vi "SelectCommand.vi"(6 "ENABLE LASER":bool=TRUE, 7 "SelectCommand":string(combo)="CharacterString", 8 "error in (no error)":errorcluster, 9 "NewString":string="Prueba", 10 "BLOK (000)":string="000", 11 "PROGRAM (0000)":string="0000") -> (0 "error out":errorcluster, 3 "Command":string="\"\"")   [LabVIEW 2018]
doc: "This VI Construct the command with the correct syntax, add new commands if is necessary here."
panel:
  in  "Counter ID":string="0"
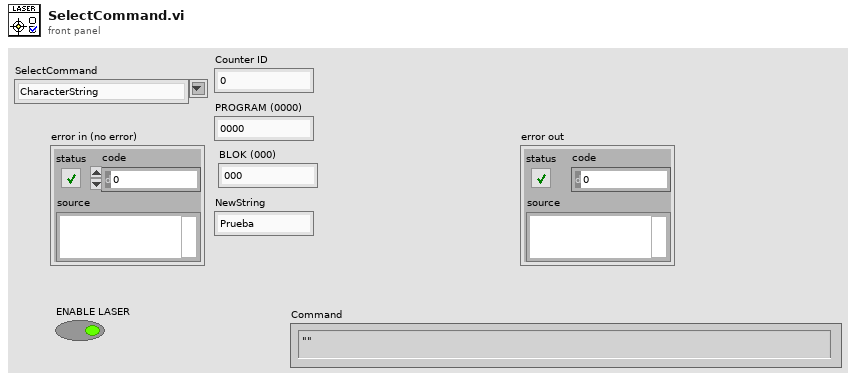
[diagram p1: front panel]
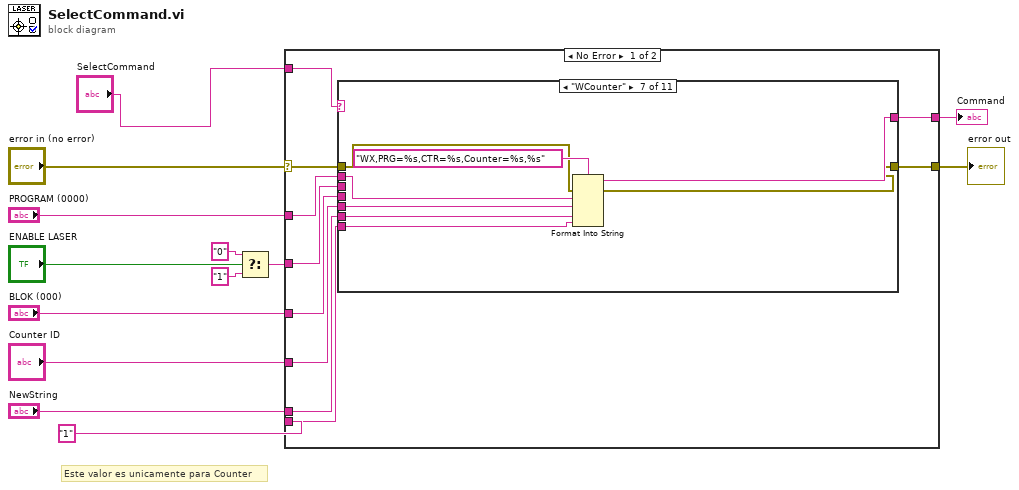
[diagram p0: block diagram]
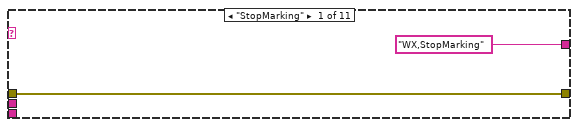
[diagram p2: hidden frame]
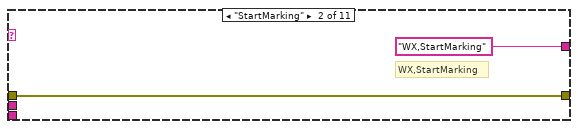
[diagram p3: hidden frame]
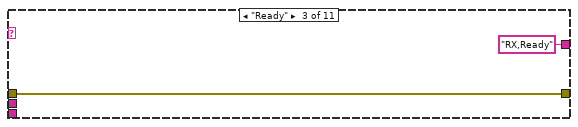
[diagram p4: hidden frame]
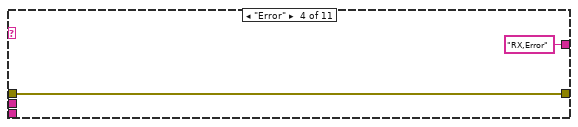
[diagram p5: hidden frame]
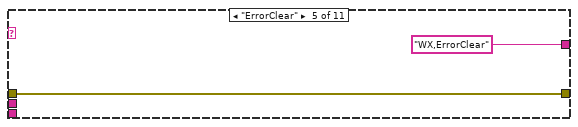
[diagram p6: hidden frame]
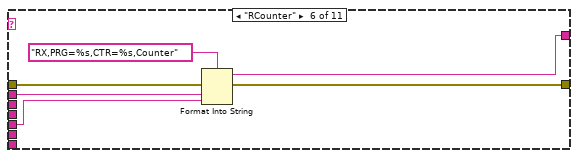
[diagram p7: hidden frame]
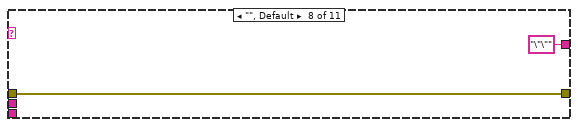
[diagram p8: hidden frame]
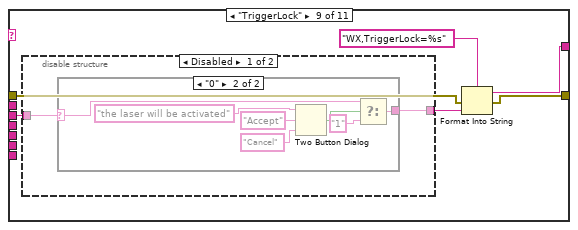
[diagram p9: hidden frame]
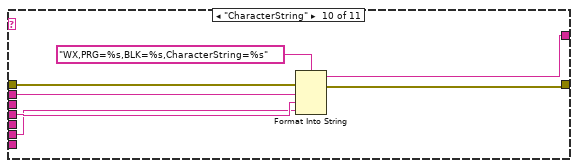
[diagram p12: hidden frame]
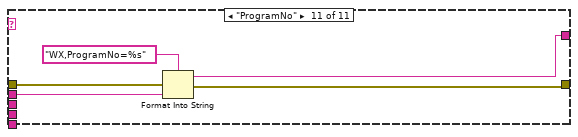
[diagram p13: hidden frame]
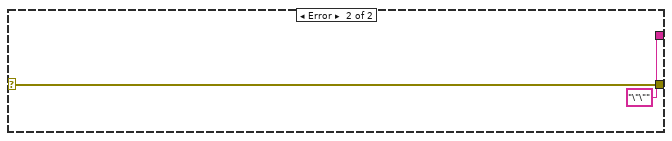
[diagram p14: hidden frame]
diagram:
  # "Este valor es unicamente para Counter"
  n1 = Select(t="0" ("WK or RX"), s="ENABLE LASER", f="1") -> (s? t:f=w4:string)
  n2 = case shown="No Error" "error in (no error)" {
    selector: "error in (no error)" -> [w16 w80]
    tunnel: [w15 w80] -> w12
    tunnel: [w23 "\"\"" ("CommandSelected")] -> w11
    tunnel: "PROGRAM (0000)" -> [w22 _]
    tunnel: "BLOK (000)" -> [w21 _]
    tunnel: "NewString" -> [w20 _]
    tunnel: w4 -> [w19 _]
    tunnel: "Counter ID" -> [w18 _]
    tunnel: "1" ("input 4") -> [w17 _]
    tunnel: "SelectCommand" -> [w14 _]
    frame No Error {
      n3 = case shown="\"WCounter\"" w14 {
        tunnel: ["WX,StopMarking" ("CommandSelected") "WX,StartMarking" ("CommandSelected") "RX,Ready" ("CommandSelected") "RX,Error" ("CommandSelected") "WX,ErrorClear" ("CommandSelected") w38 w46 "\"\"" ("CommandSelected") w55 w69 w77] -> w23
        tunnel: w22 -> [_ _ _ _ _ w37 w45 _ _ w72 w76]
        tunnel: w21 -> [_ _ _ _ _ _ _ _ _ w71 _]
        tunnel: w20 -> [_ _ _ _ _ _ w43 _ _ w70 _]
        tunnel: w19 -> [_ _ _ _ _ _ _ _ w54 _ _]
        tunnel: w18 -> [_ _ _ _ _ w36 w44 _ _ _ _]
        tunnel: w17 -> [_ _ _ _ _ _ w40 _ _ _ _]
        tunnel: w16 -> [w24 w26 w28 w30 w32 w35 w42 w48 w51 w68 w75]
        tunnel: [w24 w26 w28 w30 w32 w34 w41 w48 w50 w67 w74] -> w15
        frame "StopMarking" {
        }
        frame "StartMarking" {
          # "WX,StartMarking"
        }
        frame "Ready" {
        }
        frame "Error" {
        }
        frame "ErrorClear" {
        }
        frame "RCounter" {
          n4 = Format Into String(format string="RX,PRG=%s,CTR=%s,Counter", error in=w35, w37, w36) -> (resulting string=w38:string, error out=w34:errorcluster)  [unwired: 1 in]
        }
        frame "WCounter" {
          n5 = Format Into String(format string="WX,PRG=%s,CTR=%s,Counter=%s,%s", error in=w42, w45, w44, w43, w40) -> (resulting string=w46:string, error out=w41:errorcluster)  [unwired: 1 in]
        }
        frame "", Default {
        }
        frame "TriggerLock" {
          n6 = disable-structure shown="Disabled" {
            disable-tunnel: w54 -> [w57 w66]
            disable-tunnel: [w56 w66] -> w53
            frame Disabled {
              n7 = case shown="\"0\"" w57 {
                selector: w57 -> [w58 w61]
                tunnel: [w58 w60] -> w56
                frame "1", Default {
                }
                frame "0" {
                  n8 = Two Button Dialog(message="the laser will be activated", 1:"Cancel" ("F button name (\"Cancel\")"), 2:"Accept" ("T button name (\"OK\")")) -> (T button?=w62:bool)
                  n9 = Select(t=w61, s=w62, f="1") -> (s? t:f=w60:string)
                }
              }
            }
            frame Enabled {
            }
          }
          n10 = Format Into String(format string="WX,TriggerLock=%s", error in=w51, w53) -> (resulting string=w55:string, error out=w50:errorcluster)  [unwired: 1 in]
        }
        frame "CharacterString" {
          n11 = Format Into String(format string="WX,PRG=%s,BLK=%s,CharacterString=%s", error in=w68, w72, w71, w70) -> (resulting string=w69:string, error out=w67:errorcluster)  [unwired: 1 in]
        }
        frame "ProgramNo" {
          n12 = Format Into String(format string="WX,ProgramNo=%s", error in=w75, w76) -> (resulting string=w77:string, error out=w74:errorcluster)  [unwired: 1 in]
        }
      }
    }
    frame Error {
    }
  }
  "error out" <- w12
  "Command" <- w11
